vi "write kalman history to file.vi"(8 "error in (no error)":errorcluster, 11 "Queues":T1) -> (0 "error out":errorcluster)   [LabVIEW 2010]
uses:
  internal_queues.ctl
  line_info.ctl
  volume_with_lines.ctl
  volume_info.ctl
  kalman_result_scaled.ctl
  <vilib>/Utility/file.llb/Write To Spreadsheet File (DBL).vi
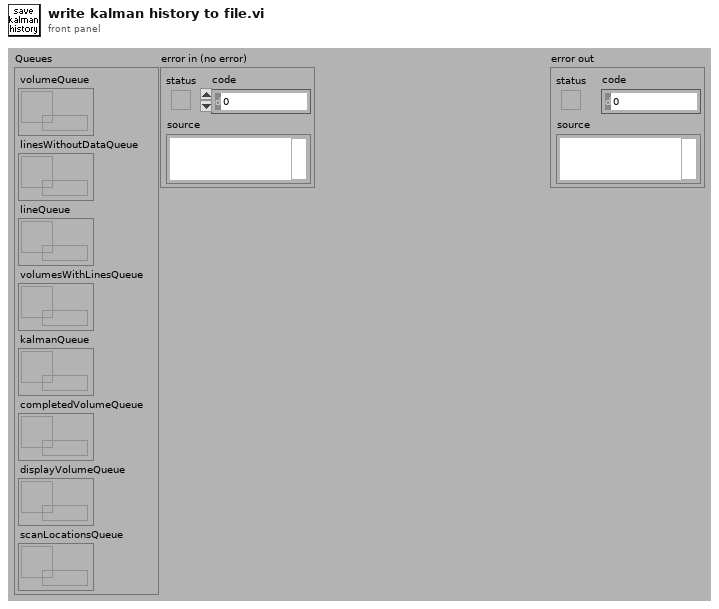
[diagram p1: front panel]
types:
  T1 = typedef "internal_queues.ctl" = cluster{"volumeQueue":refnum<queue>, "linesWithoutDataQueue":refnum<queue>, "lineQueue":refnum<queue>, "volumesWithLinesQueue":refnum<queue>, "kalmanQueue":refnum<queue>, "completedVolumeQueue":refnum<queue>, "displayVolumeQueue":refnum<queue>, "scanLocationsQueue":refnum<queue>}
  T2 = typedef "kalman_result_scaled.ctl" = cluster{"axis":u8, "pos":dbl, "vel":dbl, "p_err":dbl, "v_err":dbl, "n photon":u32, "elapsed time":dbl}
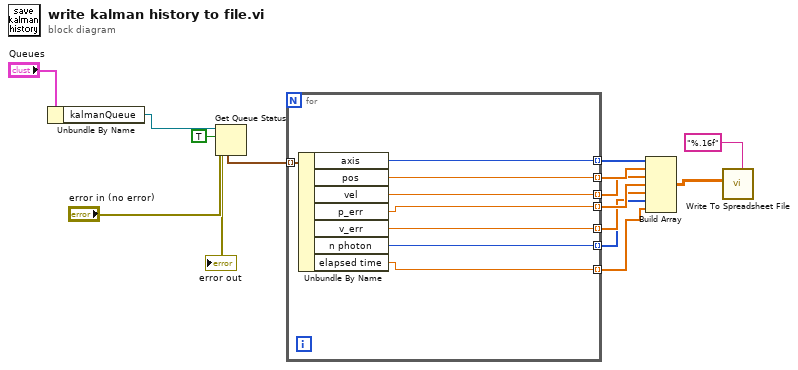
[diagram p0: block diagram]
diagram:
  n1 = Unbundle By Name("Queues") -> ("kalmanQueue"=w14:refnum<queue>)
  n2 = Get Queue Status(queue=w14, return elements? (F)=TRUE, error in (no error)="error in (no error)") -> (error out=→"error out":errorcluster, elements=w12:T2[])  [unwired: 6 out]
  n3 = for {
    tunnel: w12 -> [w23] mode=indexing
    tunnel: [w22] -> w11 mode=indexing
    tunnel: [w21] -> w10 mode=indexing
    tunnel: [w20] -> w9 mode=indexing
    tunnel: [w19] -> w8 mode=indexing
    tunnel: [w18] -> w7 mode=indexing
    tunnel: [w17] -> w6 mode=indexing
    tunnel: [w16] -> w4 mode=indexing
    n4 = Unbundle By Name(w23) -> ("axis"=w22:u8, "pos"=w21:dbl, "vel"=w20:dbl, "p_err"=w19:dbl, "v_err"=w18:dbl, "n photon"=w17:u32, "elapsed time"=w16:dbl)
  }
  n5 = Build Array(w11, w10, w9, w8, w7, w6, w4) -> (w5:dbl[][])
  n6 = call-poly <vilib>:"Write To Spreadsheet File.vi"("format (%.3f)"="%.16f", "2D data"=w5) -> ()  [unwired: 6 in, 1 out]
